vi "flip_test.vi"() -> ()   [LabVIEW 2017]
uses:
  Vision.lvlib
panel:
  in  "flip type":enum16{"Vertical", "Horizontal", "Both"}(ring)
  in  "File Path":path=path "C:/Users/Caleb/Desktop/obama.jpg"
  out "error out":errorcluster
  out "Image":T1(plugin-control)
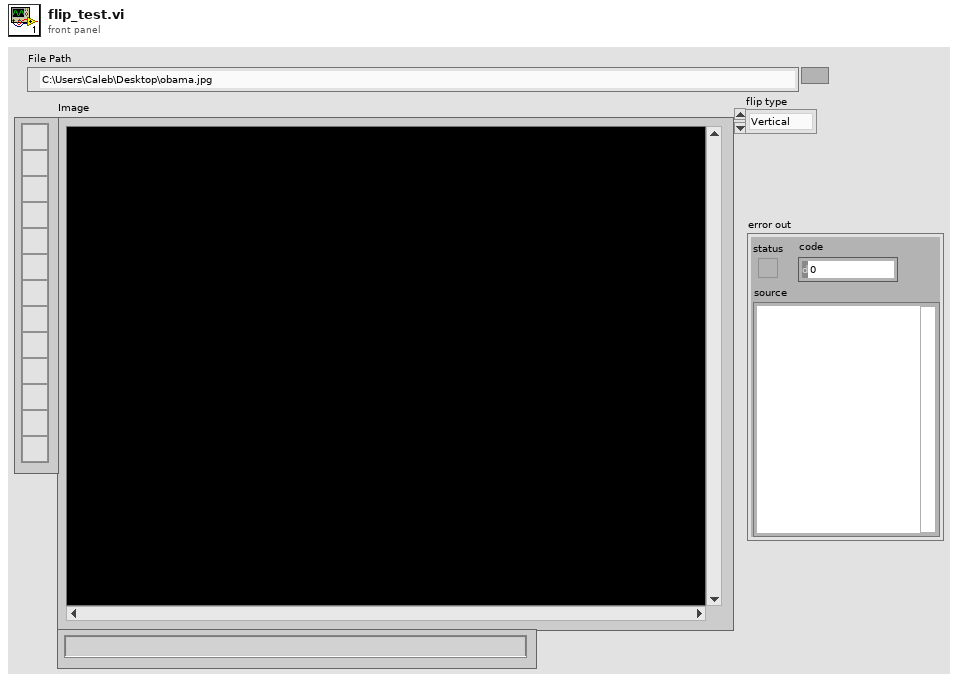
[diagram p1: front panel]
types:
  T1 = typedef "IMAQ Image.ctl" = refnum<image>
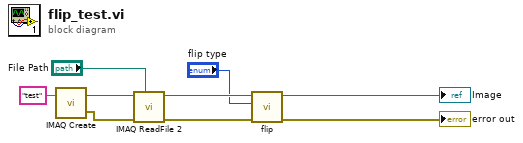
[diagram p0: block diagram]
diagram:
  n1 = call "IMAQ Create"("Image Name"="test") -> ("New Image"=w9:T1, "error out"=w7:errorcluster)  [unwired: 4 in]
  n2 = call "IMAQ ReadFile 2"("File Path"="File Path", "error in (no error)"=w7, "Image"=w9) -> ("error out"=w2:errorcluster, "Image Out"=w3:T1)  [unwired: 4 in, 3 out]
  n3 = call "flip.vi"("error in (no error)"=w2, "flip type"="flip type", "Image in"=w3) -> ("error out"=→"error out":errorcluster, "Image out"=→"Image":T1)  [unwired: 7 in]
